vi "tearDown.vi"(8 "error in (no error)":errorcluster, 11 "reference in":refnum<class "NI-SWITCH Compile Unit Tests.lvclass">) -> (0 "error out":errorcluster, 3 "reference out":refnum<class "NI-SWITCH Compile Unit Tests.lvclass">)   [LabVIEW 2017, in "NI-SWITCH Compile Unit Tests.lvclass"]
doc: "tearDown runs after the test method has completed. Use this method to clean up any operations or references that were opened by setUp or the test method. Unit tests should be independent of other unit tests so this VI should ensure that the next test can run in a 'clean' test environment."
uses:
  NI-SWITCH Compile Unit Tests.lvclass
  NI-SWITCH Compile Unit Tests.lvclass/NI-SWITCH Compile Unit Tests.ctl
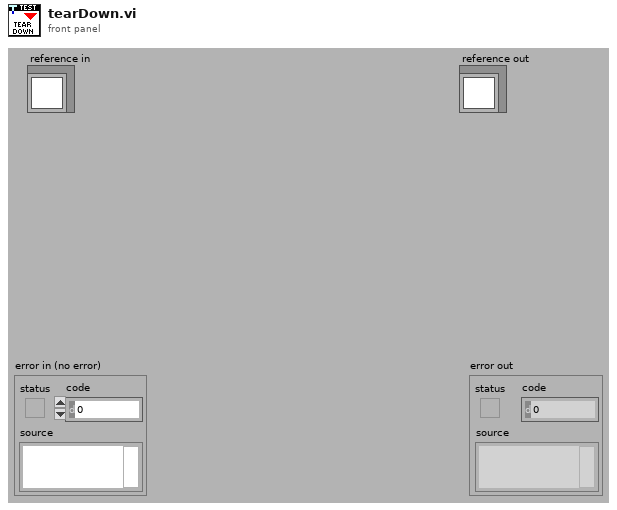
[diagram p1: front panel]
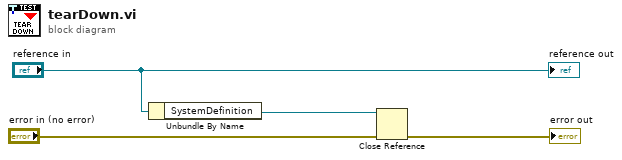
[diagram p0: block diagram]
diagram:
  n1 = Unbundle By Name("reference in") -> ("SystemDefinition"=w3:refnum<k24>)
  n2 = Close Reference(reference=w3, error in (no error)="error in (no error)") -> (error out=→"error out":errorcluster)
  "reference out" <- "reference in"
